vi "WebView2 Demo Browser (Object).vi"() -> ()   [LabVIEW 2020]
uses:
  Webview2 Lib/WebView2 Control Object/WebView2 Control.lvclass/WebView2 Control.ctl
  Webview2 Lib/WebView2 Control Object/WebView2 Control.lvclass
  Webview2 Lib/WebView2 Control Object/Paths.ctl
  C:/Users/Simon/Documents/GitHub/LV-WebView2/Source/Libs/Microsoft.Web.WebView2.WinForms.dll
  Libs/Microsoft.Web.WebView2.WinForms.dll
panel:
  out "Paths":T1
  in  "stop":bool
  in  "FWD":bool
  in  "Back":bool
  out "Status":string
  out "navigation complete":bool
  in  "Reload":bool
  in  "Go":bool
  in  "URL":string="http://ni.com"
  in  "WebView2":refnum<k24>(container)
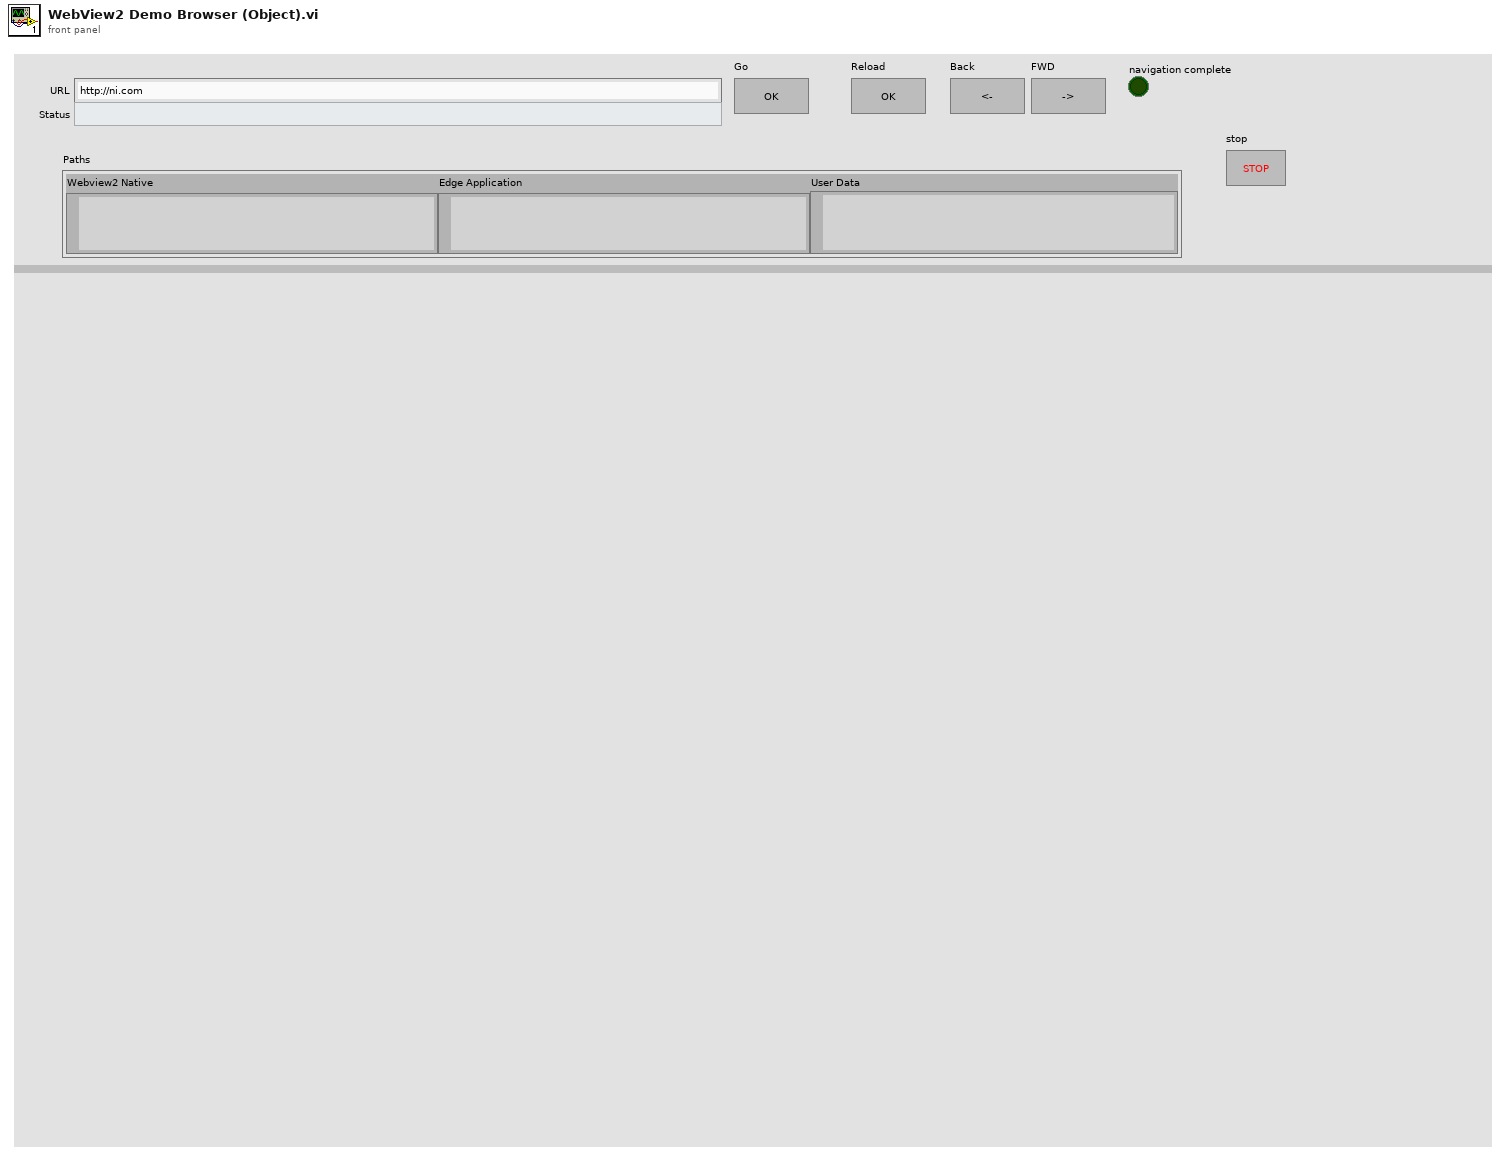
[diagram p1: front panel]
types:
  T1 = typedef "WebView2.lvlib/WebView2 Control.lvclass/Paths.ctl" = cluster{"Webview2 Native":path, "Edge Application":path, "User Data":path}
  T2 = typedef "WebView2.lvlib/WebView2 Control.lvclass/Events.ctl" = cluster{"Navigation Complete Event":refnum<user-event>, "Source Changed Event":refnum<user-event>, "Document Title Changed Event":refnum<user-event>, "Status Bar Text Changed":refnum<user-event>, "Web Message Received":refnum<user-event>, "Window Close Requested":refnum<user-event>, "DOM Loaded":refnum<user-event>, "Navigation Started Event":refnum<user-event>}
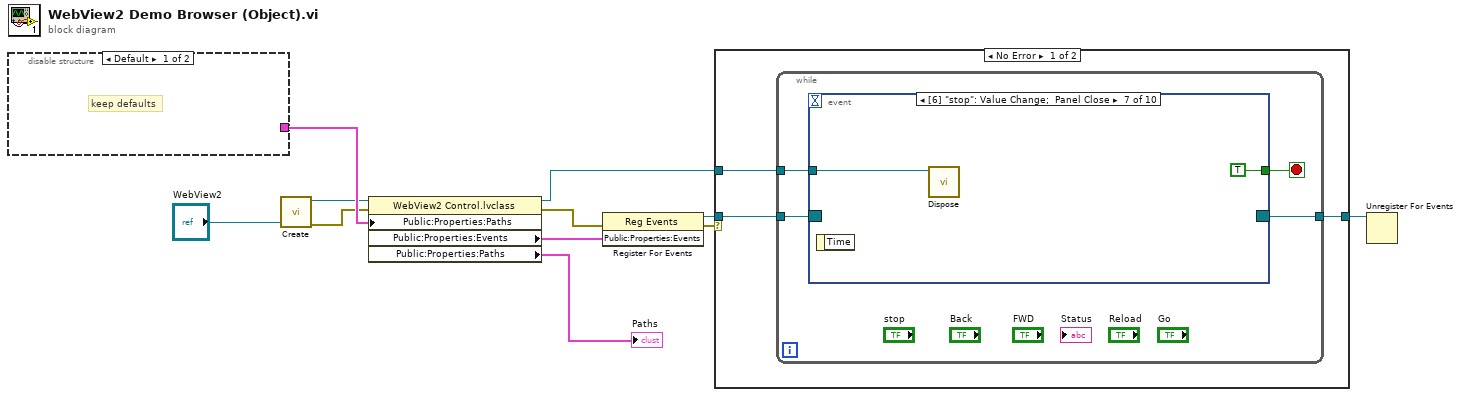
[diagram p0: block diagram]
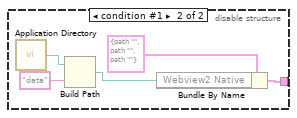
[diagram p2: hidden frame]
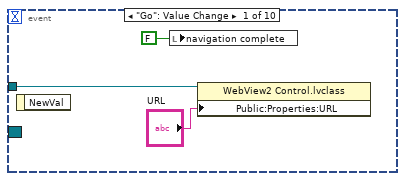
[diagram p3: hidden frame]
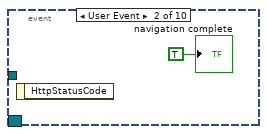
[diagram p4: hidden frame]
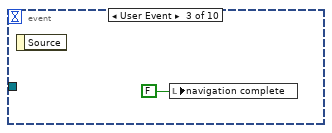
[diagram p5: hidden frame]
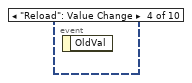
[diagram p6: hidden frame]
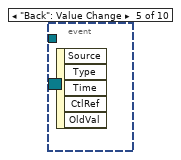
[diagram p7: hidden frame]
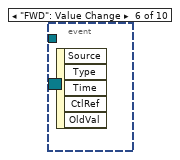
[diagram p8: hidden frame]
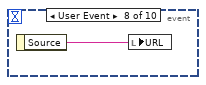
[diagram p9: hidden frame]
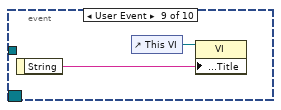
[diagram p10: hidden frame]
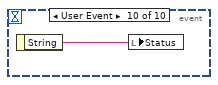
[diagram p11: hidden frame]
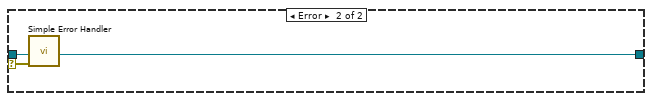
[diagram p12: hidden frame]
diagram:
  n1 = disable-structure shown="Default" {
    disable-tunnel: [_ w15] -> w5
    frame condition #0 (active) {
      # "keep defaults"
    }
    frame condition #1 {
      n2 = call <vilib>:"Application Directory.vi"() -> ("Application Directory"=w13:path)
      n3 = Build Path(base path=w13, name or relative path="data") -> (appended path=w14:path)
      n4 = Bundle By Name(cluster=T1 {"Webview2 Native"=path "", "Edge Application"=path "", "User Data"=path ""} ("Path Overrides"), "Webview2 Native"=w14) -> (w15:T1)
    }
  }
  n5 = call "Create.vi"("WebView2 Control"="WebView2") -> ("error out"=w3:errorcluster, "WebView2 Control out"=w4:refnum<class "WebView2 Control.lvclass">)  [unwired: 9 in]
  n6 = property class="WebView2 Control.lvclass"(reference=w4, error in=w3, "Public:Properties:Paths"=w5) -> (reference out=w8:refnum<class "WebView2 Control.lvclass">, error out=w6:errorcluster, "Public:Properties:Events"=w9:T2, "Public:Properties:Paths"=→"Paths":T1)
  n7 = register-events(error in=w6, w9) -> (reference out=w11:refnum<event-registration>, error out=w10:errorcluster)  [unwired: 1 in]
  n8 = case shown="No Error" w10 {
    selector: w10 -> [_ w36]
    tunnel: w11 -> [w19 w35]
    tunnel: w8 -> [w18 _]
    tunnel: [w17 w35] -> w7
    frame No Error {
      n9 = while {
        tunnel: w19 -> [w23]
        tunnel: w18 -> [w21]
        tunnel: [w20] -> w17
        stop <- w22 stop-if-true
        n10 = event shown="[6] \"stop\": Value Change;  Panel Close" {
          selector: w23 -> [_ _ _ _ _ _ _ _ _ _]
          dyn-events: [_ _ _ _ _ _ _ _ _ _] -> w20
          timeout: _ -> [_ _ _ _ _ _ _ _ _ _]
          tunnel: [_ _ _ _ _ _ TRUE _ _ _] -> w22
          tunnel: w21 -> [w25 _ _ _ _ _ w29 _ _ _]
          event "Go": Value Change {
            n11 = event-data() -> ()  [unwired: 1 in, 1 out]
            n12 = local write "navigation complete"(FALSE ("navigation complete")) -> ()
            n13 = property class="WebView2 Control.lvclass"(reference=w25, "Public:Properties:URL"="URL") -> ()  [unwired: 1 in, 2 out]
          }
          event User Event {
            n14 = event-data() -> ()  [unwired: 1 in, 1 out]
            "navigation complete" <- TRUE ("navigation complete")
          }
          event User Event {
            n15 = event-data() -> ()  [unwired: 1 in, 1 out]
            n16 = local write "navigation complete"(FALSE ("navigation complete")) -> ()
          }
          event "Reload": Value Change {
            n17 = event-data() -> ()  [unwired: 1 in, 1 out]
          }
          event "Back": Value Change {
            n18 = event-data() -> ()  [unwired: 1 in, 5 out]
          }
          event "FWD": Value Change {
            n19 = event-data() -> ()  [unwired: 1 in, 5 out]
          }
          event "stop": Value Change; Panel Close {
            n20 = event-data() -> ()  [unwired: 1 in, 1 out]
            n21 = call "Dispose.vi"("WebView2 Control in"=w29) -> ()  [unwired: 10 in, 1 out]
          }
          event User Event {
            n22 = event-data() -> ("Source"=w31:string)  [unwired: 1 in]
            n23 = local write "URL"(w31) -> ()
          }
          event User Event {
            n24 = event-data() -> ("String"=w32:string)  [unwired: 1 in]
            n25 = control-ref of="This VI"() -> (w33:refnum<vi>)
            n26 = property class="VI"(reference=w33, "Front Panel.Title"=w32) -> ()  [unwired: 1 in, 2 out]
          }
          event User Event {
            n27 = event-data() -> ("String"=w34:string)  [unwired: 1 in]
            n28 = local write "Status"(w34) -> ()
          }
        }
      }
    }
    frame Error {
      n29 = call <vilib>:"Simple Error Handler.vi"("error in (no error)"=w36) -> ()  [unwired: 4 in, 5 out]
    }
  }
  n30 = Unregister For Events(event registration refnum=w7) -> ()  [unwired: 1 in, 1 out]
